vi "Not A Rendezvous.vi"(1 "rendezvous":T1) -> (0 "not a rendezvous":bool)   [LabVIEW 2010]
doc: "Returns TRUE if <B>rendezvous</B> is not a valid rendezvous refnum."
uses:
  RendezvousDataCluster.ctl
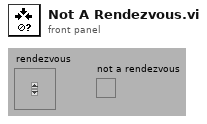
[diagram p1: front panel]
types:
  T1 = typedef "Rendezvous RefNum" = refnum<k1>
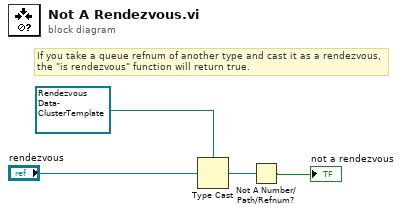
[diagram p0: block diagram]
diagram:
  # "If you take a queue refnum of another type and cast it as a rendezvous,\nthe \"is rendezvous\" function will return true."
  n1 = Type Cast(type=refnum<queue> refnum ("queue out"), x="rendezvous") -> (*(type *) &x=w4:refnum<queue>)
  n2 = Not A Number/Path/Refnum?(number/path/refnum=w4) -> (NaN/Path/Refnum?=→"not a rendezvous":bool)
